vi "PRL Read Buffer Private.vi"(0 "Read":bool, 1 "Get All Signals":bool, 2 "Initialize In":bool, 5 "Get Full Buffer?":bool, 12 "Time  Stamp In":timestamp) -> (3 "Initialize Out":bool, 4 "Timestamp":timestamp[](array[timestamp]), 6 "Phasor Signals":csg[][](array[numeric]), 10 "Analog Signals":sgl[][](array[numeric]), 11 "Has Data?":bool, 13 "First Buffer Filled":bool, 14 "Time Stamp Out":timestamp, 15 "Digital Signals":bool[][](array[boolean]))   [LabVIEW 2017, in "PMU Recorder Light.lvlib"]
doc: "Reads the newest data from the PRL Accsess Buffer."
uses:
  PMU Recorder Light.lvlib
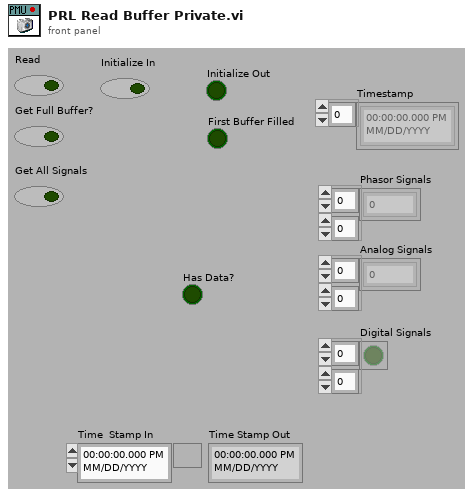
[diagram p1: front panel]
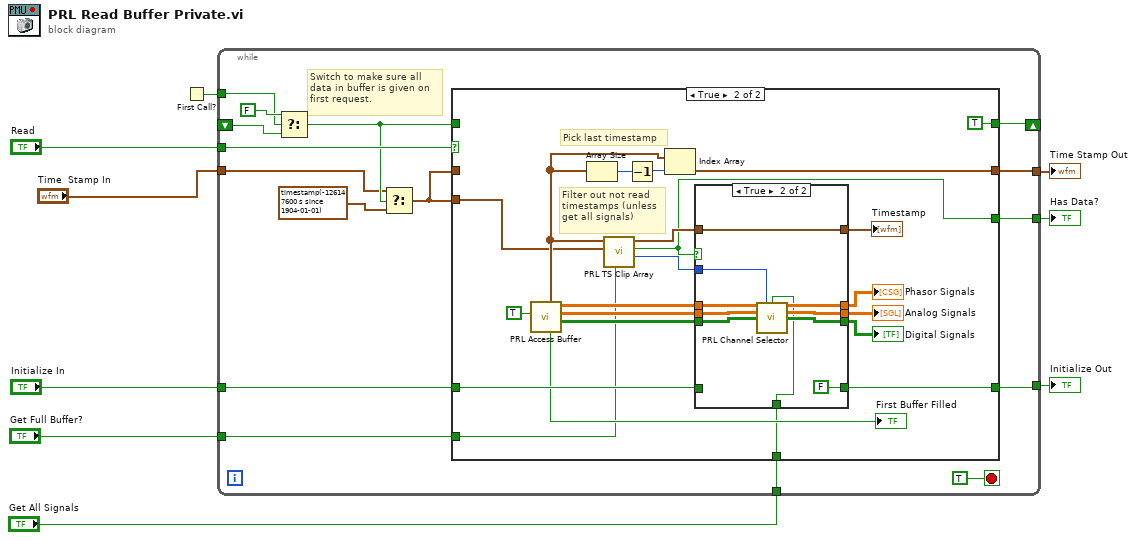
[diagram p0: block diagram]
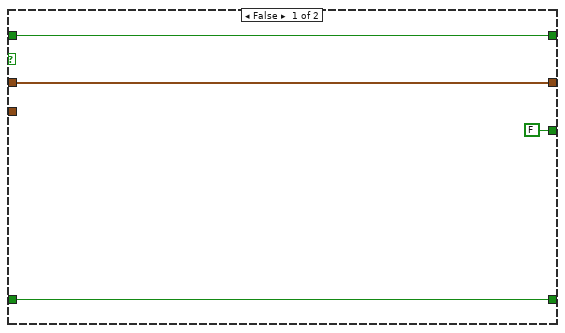
[diagram p2: hidden frame]
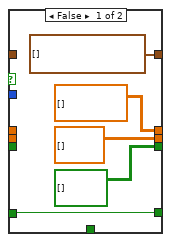
[diagram p3: hidden frame]
diagram:
  n1 = First Call?() -> (First Call?: T/F=w9:bool)
  n2 = while {
    tunnel: w9 -> [w21]
    tunnel: "Read" -> [w24]
    shift-right: [w20] -> _
    shift-left: _ -> [w22]
    tunnel: "Initialize In" -> [w19]
    tunnel: "Get Full Buffer?" -> [w18]
    tunnel: [w17] -> w5
    tunnel: "Time  Stamp In" -> [w11]
    tunnel: [w16] -> w3
    tunnel: [w15] -> w2
    tunnel: "Get All Signals" -> [w14]
    stop <- TRUE stop-if-true
    # "Switch to make sure all\ndata in buffer is given on\nfirst request."
    n3 = Select(t=FALSE ("First Call?: T/F"), s=w21, f=w22) -> (s? t:f=w13:bool)
    n4 = Select(t=w11, s=w13, f=timestamp(-126147600 s since 1904-01-01) ("Time  Stamp In")) -> (s? t:f=w10:timestamp)
    n5 = case shown="True" w24 {
      tunnel: [w29 w49] -> w16
      tunnel: w10 -> [w29 _]
      tunnel: w13 -> [w28 _]
      tunnel: [w28 TRUE ("First Call?: T/F")] -> w20
      tunnel: w19 -> [w27 w46]
      tunnel: w18 -> [_ w33]
      tunnel: [w27 w44] -> w17
      tunnel: [FALSE ("Has Data?") w35] -> w15
      tunnel: w14 -> [_ w32]
      tunnel: w10 -> [_ w31]
      frame False {
      }
      frame True {
        # "Filter out not read\ntimestamps (unless\nget all signals)"
        # "Pick last timestamp"
        n6 = call "PRL Access Buffer.vi"("Read Data?"=TRUE) -> ("Digital Values"=w40:bool[][], "Analog Values"=w42:sgl[][], "Phasor Values"=w43:csg[][], "First Buffer Filled"=→"First Buffer Filled":bool, "Timestamp Values"=w41:timestamp[])  [unwired: 4 in, 2 out]
        n7 = Array Size(array=w41) -> (size(s)=w51:i32)
        n8 = call "PRL TS Clip Array.vi"("Get Full Buffer"=w33, "Start Timestamp"=w31, "Timestamp In"=w41) -> ("Index"=w47:i32, "Has Data?"=w35:bool, "Timestamp Out"=w45:timestamp[])  [unwired: 6 in]
        n9 = Decrement(x=w51) -> (x-1=w50:i32)
        n10 = Index Array(array=w41, index=w50) -> (element=w49:timestamp)
        n11 = case shown="True" w35 {
          tunnel: w47 -> [_ w59]
          tunnel: w43 -> [_ w65]
          tunnel: w42 -> [_ w64]
          tunnel: w46 -> [w56 _]
          tunnel: w45 -> [_ w57]
          tunnel: [w56 FALSE ("First Call?: T/F")] -> w44
          tunnel: w40 -> [_ w63]
          tunnel: [csg[][] [] ("Phasor Signals") w62] -> w38
          tunnel: [sgl[][] [] ("Analog Signals") w61] -> w37
          tunnel: [bool[][] [] ("Digital Signals") w60] -> w36
          tunnel: w32 -> [_ w58]
          tunnel: [timestamp[] [] ("Timestamp Out") w57] -> w30
          frame False {
          }
          frame True {
            n12 = call "PRL Channel Selector.vi"("Phasor Values In"=w65, "Cut Index"=w59, "Get All Signals"=w58, "Analog Values In"=w64, "Digital Values In"=w63) -> ("Phasor Values Out"=w62:csg[][], "Analog Values Out"=w61:sgl[][], "Digital Values Out"=w60:bool[][])  [unwired: 7 in, 1 out]
          }
        }
        "Phasor Signals" <- w38
        "Analog Signals" <- w37
        "Digital Signals" <- w36
        "Timestamp" <- w30
      }
    }
  }
  "Initialize Out" <- w5
  "Time Stamp Out" <- w3
  "Has Data?" <- w2
